vi "phase_tracking.vi"() -> ()   [LabVIEW 2017]
uses:
  <vilib>/rvi/FXPMathLib/FxpSinAndCos/subVIs/nifxpmath_SinAndCos_SimConfig.ctl
  <vilib>/rvi/FXPMathLib/FxpAtan2/subVIs/nifxpmath_Atan2_SimConfig.ctl
  <vilib>/rvi/Emulation/niFpgaGetClockAttributes.vi
  <vilib>/rvi/Emulation/niFpgaSctlEmulationGetInTimedLoop.vi
  <vilib>/rvi/Emulation/niFpgaEmulationReportErrorSimple.vi
  <vilib>/rvi/eio/common/nirviEmuTemplateMethod_errors.vi
  <vilib>/rvi/FXPMathLib/FxpSinAndCos/simVIs/DllFxpSinAndCosTemp_sub.vi
  <vilib>/rvi/FXPMathLib/FxpAtan2/simVIs/DllFxpAtan2Temp_sub.vi
  <vilib>/rvi/Emulation/niFpgaCriticalErrorInLSC.vi
  <vilib>/eio/EIONode/EIONode.xnode
  <vilib>/rvi/Analysis/measure/butterworth/XNode/niFpgaButterworthFilter.xnode
  <vilib>/rvi/FXPMathLib/FxpSinAndCos/XNode/nifxpmath_SinAndCos.xnode
  <vilib>/rvi/FXPMathLib/basic elements/FxpDiscreteDelay/XNode/nifxpmath_DiscreteDelay.xnode
  <vilib>/rvi/FXPMathLib/FxpAtan2/XNode/nifxpmath_Atan2.xnode
panel:
  in  "phase_filt_coeffs":i32[](array[numeric])=[0, 0, 0, 0, 0, 0]
  out "Phi Full":fxp<+/-,32,18>=2.0 format="%.20g"
  out "n":i16
  out "Phi":fxp<+/-,16,2>
  in  "delay":u16
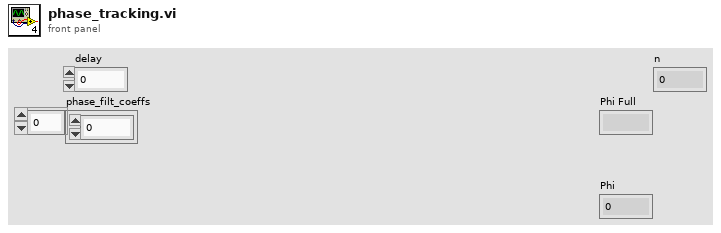
[diagram p1: front panel]
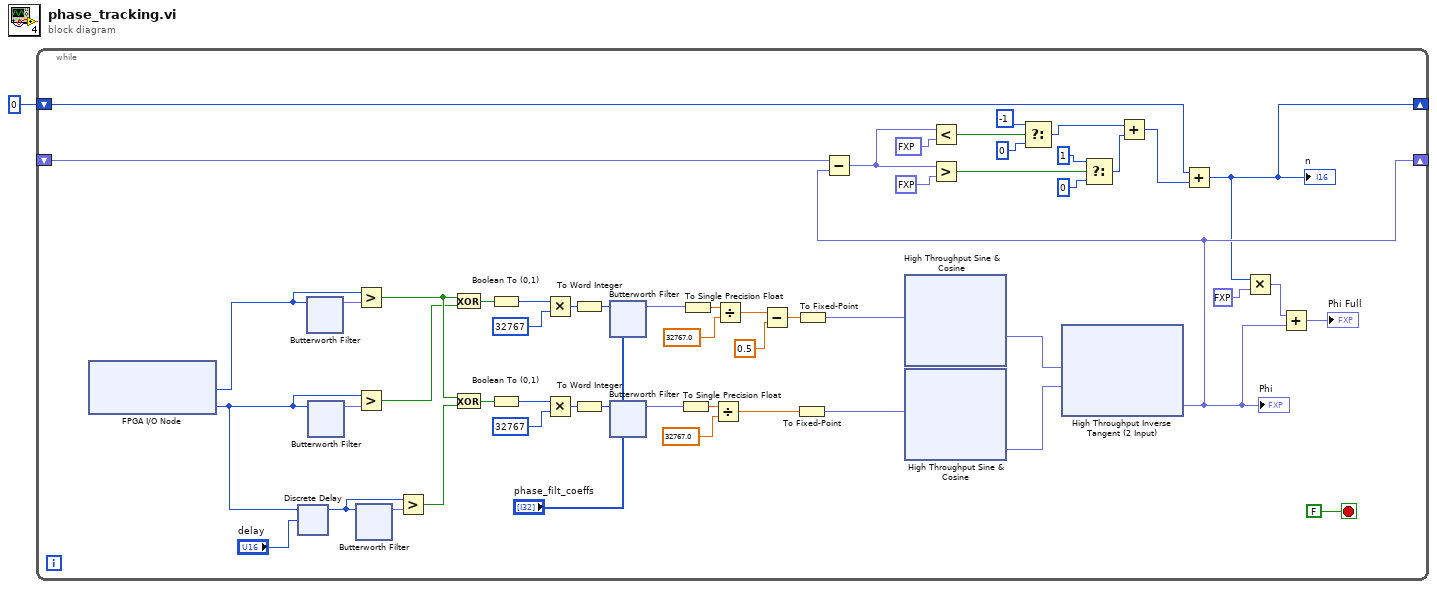
[diagram p0: block diagram]
diagram:
  n1 = while {
    shift-right: [w3] -> _
    shift-left: i16 0 -> [w10]
    shift-right: [w6] -> _
    shift-left: _ -> [w9]
    stop <- FALSE stop-if-true
    n2 = xnode "FPGA I/O Node"() -> ("Connector0/AI0"=w53:i16, "Connector0/AI1"=w38:i16)  [unwired: 2 in, 2 out]
    n3 = xnode ("Discrete Delay")("D"=w38, "n-1[0..511]"="delay") -> ("Q"=w37:i16)
    n4 = xnode "Butterworth Filter"("input data"=w53) -> ("output data"=w55:fxp<+/-,20,20>)  [unwired: 2 in]
    n5 = xnode "Butterworth Filter"("input data"=w38) -> ("output data"=w54:fxp<+/-,20,20>)  [unwired: 2 in]
    n6 = Greater?(x=w53, y=w55) -> (0:w41:bool)
    n7 = Greater?(x=w38, y=w54) -> (0:w40:bool)
    n8 = xnode "Butterworth Filter"("input data"=w37) -> ("output data"=w52:fxp<+/-,20,20>)  [unwired: 2 in]
    n9 = Greater?(x=w37, y=w52) -> (0:w39:bool)
    n10 = Exclusive Or(1:w40, 2:w41) -> (0:w51:bool)
    n11 = Exclusive Or(1:w39, 2:w41) -> (0:w46:bool)
    n12 = Boolean To (0,1)(Boolean=w51) -> (0, 1=w49:i16)
    n13 = Boolean To (0,1)(Boolean=w46) -> (0, 1=w44:i16)
    n14 = Multiply(x=w49, y=i16 32767) -> (x*y=w48:i16)
    n15 = Multiply(x=w44, y=i16 32767) -> (x*y=w43:i16)
    n16 = To Word Integer(number=w48) -> (16bit integer=w50:i16)
    n17 = To Word Integer(number=w43) -> (16bit integer=w45:i16)
    n18 = xnode "Butterworth Filter"("input data"=w50, "scaled coefficients"="phase_filt_coeffs") -> ("output data"=w35:fxp<+/-,20,20>)  [unwired: 1 in]
    n19 = xnode "Butterworth Filter"("input data"=w45, "scaled coefficients"="phase_filt_coeffs") -> ("output data"=w31:fxp<+/-,20,20>)  [unwired: 1 in]
    n20 = To Single Precision Float(number=w31) -> (single precision float=w33:sgl)
    n21 = To Single Precision Float(number=w35) -> (single precision float=w36:sgl)
    n22 = Divide(x=w33, y=sgl 32767.0) -> (x/y=w8:sgl)
    n23 = Divide(x=w36, y=sgl 32767.0) -> (x/y=w29:sgl)
    n24 = Subtract(x=w29, y=sgl 0.5 ("sin sub")) -> (x-y=w27:sgl)
    n25 = To Fixed-Point(number=w8) -> (fixed-point=w23:fxp<+/-,32,16>)  [unwired: 1 in]
    n26 = To Fixed-Point(number=w27) -> (fixed-point=w30:fxp<+/-,32,16>)  [unwired: 1 in]
    n27 = xnode "High Throughput Sine & Cosine"("x (pi)"=w30) -> ("sin(x)"=w26:fxp<+/-,16,2>)  [unwired: 1 out]
    n28 = xnode "High Throughput Sine & Cosine"("x (pi)"=w23) -> ("cos(x)"=w24:fxp<+/-,16,2>)  [unwired: 1 out]
    n29 = xnode "High Throughput Inverse Tangent (2 Input)"("y"=w26, "x"=w24) -> ("atan2(y,x) (pi)"=w6:fxp<+/-,16,2>)
    "Phi" <- w6
    n30 = Subtract(x=w9, y=w6) -> (x-y=w21:fxp<+/-,17,3>)
    n31 = Less?(x=w21, y=fxp<+/-,3,2> -1.5) -> (x < y?=w18:bool)
    n32 = Greater?(x=w21, y=fxp<+,2,1> 1.5) -> (0:w14:bool)
    n33 = Select(t=i16 -1, s=w18, f=i16 0) -> (s? t:f=w13:i16)
    n34 = Select(t=i16 1, s=w14, f=i16 0) -> (s? t:f=w12:i16)
    n35 = Add(x=w13, y=w12) -> (x+y=w11:i16)
    n36 = Add(x=w10, y=w11) -> (x+y=w3:i16)
    "n" <- w3
    n37 = Multiply(x=w3, y=fxp<+,1,2> 2.0) -> (x*y=w5:fxp<+/-,16,17>)
    n38 = Add(x=w5, y=w6) -> (x+y=→"Phi Full":fxp<+/-,32,18>)
  }
